vi "sbRIO Example.vi"() -> ()   [LabVIEW 2012]
uses:
  <vilib>/rvi/interface/RandomDataEmulation/nirviRandomDataFPGAFIFO.vi
  <vilib>/rvi/interface/RandomDataEmulation/niFpgaRandomDataHandleErrors.vi
  <vilib>/rvi/DataTransferAndStorage/Container/XNode/niFpgaContainer.xnode
  <vilib>/rvi/interface/RandomDataEmulation/nirviRandomDataFpgaReadWriteTemplate.vi
  UART 8N1 (FPGA).lvlib
panel:
  in  "stop":bool
  out "Read Data":u8
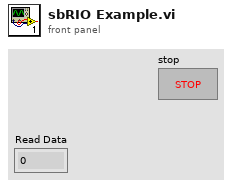
[diagram p1: front panel]
types:
  T1 = cluster{"Stop Ref":refnum<k21>, "Buffer Ref":refnum<k21>}
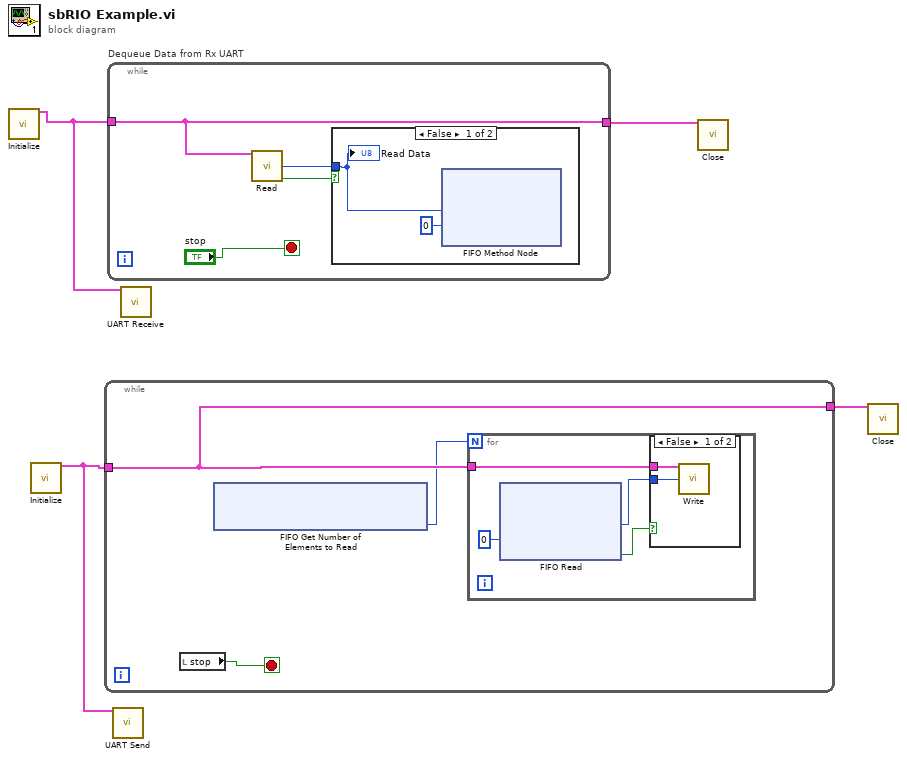
[diagram p0: block diagram]
diagram:
  n1 = call "Initialize.vi"() -> ("I/O Out"=w1:T1)  [unwired: 15 in]
  n2 = call "Initialize.vi"() -> ("I/O Out"=w4:T1)  [unwired: 15 in]
  n3 = while {
    tunnel: w4 -> [w6]
    tunnel: [w6] -> w2
    stop <- w7 stop-if-true
    n4 = local read "stop"() -> (w7:bool)
    n5 = xnode "FIFO Get Number of Elements to Read"() -> ("Number of Elements to Read"=w5:u32)  [unwired: 1 in, 1 out]
    n6 = for {
      N: w5 -> [_]
      tunnel: w6 -> [w11]
      n7 = xnode "FIFO Read"("Timeout"=0) -> ("Element"=w9:u8, "Timed Out?"=w8:bool)  [unwired: 1 in, 1 out]
      n8 = case shown="False" w8 {
        tunnel: w11 -> [w13 _]
        tunnel: w9 -> [w12 _]
        frame False {
          n9 = call "Write.vi"("I/O In"=w13, "Data"=w12) -> ()  [unwired: 12 in, 2 out]
        }
        frame True {
        }
      }
    }
  }
  n10 = while "Dequeue Data from Rx UART" {
    tunnel: w1 -> [w14]
    tunnel: [w14] -> w3
    stop <- "stop" stop-if-true
    n11 = call "Read.vi"("I/O In"=w14) -> ("Data"=w17:u8, "Timed Out?"=w16:bool)  [unwired: 12 in, 1 out]
    n12 = case shown="False" w16 {
      tunnel: w17 -> [w19 _]
      frame False {
        n13 = xnode ("FIFO Method Node")("Element"=w19, "Timeout"=0) -> ()  [unwired: 1 in, 2 out]
        "Read Data" <- w19
      }
      frame True {
      }
    }
  }
  n14 = call "UART Send.vi"("I/O In"=w4) -> ()  [unwired: 15 in]
  n15 = call "UART Receive.vi"("I/O In"=w1) -> ()  [unwired: 14 in, 1 out]
  n16 = call "Close.vi"("I/O In"=w3) -> ()  [unwired: 15 in]
  n17 = call "Close.vi"("I/O In"=w2) -> ()  [unwired: 15 in]
